vi "Day 14 - Part two.vi"() -> ()   [LabVIEW 2025]
panel:
  out "i":i32
  out "# of sand":i32
  out "cave array":string[][](array[string])
  out "lines array":string[](array[string])
  out "sand pour":i32
  out "Y offset":i32
  out "X":i32
  out "Y":i32
  in  "test":bool
  in  "test input":string="498,4 -> 498,6 -> 496,6\n503,4 -> 502,4 -> 502,9 -> 494,9"
  in  "input":string="487,45 -> 487,38 -> 487,45 -> 489,45 -> 489,42 -> 489,45 -> 491,45 -> 491,39 -> 491,45 -> 493,45 -> 493,39 -> 493,45\n512,90 -> 512,87 -> 512,90 -> 514,90 -> 514,86 -> 514,90 -> 516,90 -> 516,87 -> 516,90 -> 518,90 -> 518,82 -> 518,90 -> 520,90 -> 520,81 -> 520,90 -> 522,90 -> 522,86 -> 522,90 -> 524,90 -> 524,84 -> 524,90 -> 526,90 -> 526,82 -> 526,90 -> 528,90 -> 528,82 -> 528,90\n494,16 -> 499,16\n512,90 -> 512,87 -> 512,90 -> 514,90 -> 514,86 -> 514,90 -> 516,90 -> 516,87 -> 516,90 -> 518,90 -> 518,82 -> 518,90 -> 520,90 -> 520,81 -> 520,90 -> 522,90 -> 522,86 -> 522,90 -> 524,90 -> 524,84 -> 524,90 -> 526,90 -> 526,82 -> 526,90 -> 528,90 -> 528,82 -> 528,90\n505,57 -> 505,59 -> 498,59 -> 498,66 -> 509,66 -> 509,59 -> 507,59 -> 507,57\n492,52 -> 496,52\n520,165 -> 520,160 -> 520,165 -> 522,165 -> 522,163 -> 522,165 -> 524,165 -> 524,159 -> 524,165 -> 526,165 -> 526,159 -> 526,165 -> 528,165 -> 528,155 -> 528,165\n510,123 -> 515,123\n492,48 -> 496,48\n512,90 -> 512,87 -> 512,90 -> 514,90 -> 514,86 -> 514,90 -> 516,90 -> 516,87 -> 516,90 -> 518,90 -> 518,82 -> 518,90 -> 520,90 -> 520,81 -> 520,90 -> 522,90 -> 522,86 -> 522,90 -> 524,90 -> 524,84 -> 524,90 -> 526,90 -> 526,82 -> 526,90 -> 528,90 -> 528,82 -> 528,90\n512,90 -> 512,87 -> 512,90 -> 514,90 -> 514,86 -> 514,90 -> 516,90 -> 516,87 -> 516,90 -> 518,90 -> 518,82 -> 518,90 -> 520,90 -> 520,81 -> 520,90 -> 522,90 -> 522,86 -> 522,90 -> 524,90 -> 524,84 -> 524,90 -> 526,90 -> 526,82 -> 526,90 -> 528,90 -> 528,82 -> 528,90\n487,45 -> 487,38 -> 487,45 -> 489,45 -> 489,42 -> 489,45 -> 491,45 -> 491,39 -> 491,45 -> 493,45 -> 493,39 -> 493,45\n501,54 -> 505,54\n513,120 -> 518,120\n502,138 -> 502,141 -> 498,141 -> 498,145 -> 514,145 -> 514,141 -> 507,141 -> 507,138\n483,54 -> 487,54\n505,57 -> 505,59 -> 498,59 -> 498,66 -> 509,66 -> 509,59 -> 507,59 -> 507,57\n508,103 -> 508,93 -> 508,103 -> 510,103 -> 510,101 -> 510,103 -> 512,103 -> 512,96 -> 512,103\n512,106 -> 512,108 -> 505,108 -> 505,114 -> 518,114 -> 518,108 -> 516,108 -> 516,106\n532,129 -> 537,129\n501,16 -> 506,16\n508,103 -> 508,93 -> 508,103 -> 510,103 -> 510,101 -> 510,103 -> 512,103 -> 512,96 -> 512,103\n502,138 -> 502,141 -> 498,141 -> 498,145 -> 514,145 -> 514,141 -> 507,141 -> 507,138\n520,120 -> 525,120\n489,50 -> 493,50\n498,19 -> 503,19\n505,151 -> 505,152 -> 518,152 -> 518,151\n510,73 -> 514,73\n516,77 -> 520,77\n487,45 -> 487,38 -> 487,45 -> 489,45 -> 489,42 -> 489,45 -> 491,45 -> 491,39 -> 491,45 -> 493,45 -> 493,39 -> 493,45\n520,165 -> 520,160 -> 520,165 -> 522,165 -> 522,163 -> 522,165 -> 524,165 -> 524,159 -> 524,165 -> 526,165 -> 526,159 -> 526,165 -> 528,165 -> 528,155 -> 528,165\n512,90 -> 512,87 -> 512,90 -> 514,90 -> 514,86 -> 514,90 -> 516,90 -> 516,87 -> 516,90 -> 518,90 -> 518,82 -> 518,90 -> 520,90 -> 520,81 -> 520,90 -> 522,90 -> 522,86 -> 522,90 -> 524,90 -> 524,84 -> 524,90 -> 526,90 -> 526,82 -> 526,90 -> 528,90 -> 528,82 -> 528,90\n511,129 -> 516,129\n512,90 -> 512,87 -> 512,90 -> 514,90 -> 514,86 -> 514,90 -> 516,90 -> 516,87 -> 516,90 -> 518,90 -> 518,82 -> 518,90 -> 520,90 -> 520,81 -> 520,90 -> 522,90 -> 522,86 -> 522,90 -> 524,90 -> 524,84 -> 524,90 -> 526,90 -> 526,82 -> 526,90 -> 528,90 -> 528,82 -> 528,90\n520,165 -> 520,160 -> 520,165 -> 522,165 -> 522,163 -> 522,165 -> 524,165 -> 524,159 -> 524,165 -> 526,165 -> 526,159 -> 526,165 -> 528,165 -> 528,155 -> 528,165\n512,90 -> 512,87 -> 512,90 -> 514,90 -> 514,86 -> 514,90 -> 516,90 -> 516,87 -> 516,90 -> 518,90 -> 518,82 -> 518,90 -> 520,90 -> 520,81 -> 520,90 -> 522,90 -> 522,86 -> 522,90 -> 524,90 -> 524,84 -> 524,90 -> 526,90 -> 526,82 -> 526,90 -> 528,90 -> 528,82 -> 528,90\n524,123 -> 529,123\n512,90 -> 512,87 -> 512,90 -> 514,90 -> 514,86 -> 514,90 -> 516,90 -> 516,87 -> 516,90 -> 518,90 -> 518,82 -> 518,90 -> 520,90 -> 520,81 -> 520,90 -> 522,90 -> 522,86 -> 522,90 -> 524,90 -> 524,84 -> 524,90 -> 526,90 -> 526,82 -> 526,90 -> 528,90 -> 528,82 -> 528,90\n505,57 -> 505,59 -> 498,59 -> 498,66 -> 509,66 -> 509,59 -> 507,59 -> 507,57\n487,45 -> 487,38 -> 487,45 -> 489,45 -> 489,42 -> 489,45 -> 491,45 -> 491,39 -> 491,45 -> 493,45 -> 493,39 -> 493,45\n520,165 -> 520,160 -> 520,165 -> 522,165 -> 522,163 -> 522,165 -> 524,165 -> 524,159 -> 524,165 -> 526,165 -> 526,159 -> 526,165 -> 528,165 -> 528,155 -> 528,165\n512,90 -> 512,87 -> 512,90 -> 514,90 -> 514,86 -> 514,90 -> 516,90 -> 516,87 -> 516,90 -> 518,90 -> 518,82 -> 518,90 -> 520,90 -> 520,81 -> 520,90 -> 522,90 -> 522,86 -> 522,90 -> 524,90 -> 524,84 -> 524,90 -> 526,90 -> 526,82 -> 526,90 -> 528,90 -> 528,82 -> 528,90\n507,75 -> 511,75\n495,22 -> 495,25 -> 492,25 -> 492,32 -> 501,32 -> 501,25 -> 499,25 -> 499,22\n514,149 -> 524,149 -> 524,148\n512,90 -> 512,87 -> 512,90 -> 514,90 -> 514,86 -> 514,90 -> 516,90 -> 516,87 -> 516,90 -> 518,90 -> 518,82 -> 518,90 -> 520,90 -> 520,81 -> 520,90 -> 522,90 -> 522,86 -> 522,90 -> 524,90 -> 524,84 -> 524,90 -> 526,90 -> 526,82 -> 526,90 -> 528,90 -> 528,82 -> 528,90\n504,129 -> 509,129\n487,45 -> 487,38 -> 487,45 -> 489,45 -> 489,42 -> 489,45 -> 491,45 -> 491,39 -> 491,45 -> 493,45 -> 493,39 -> 493,45\n520,165 -> 520,160 -> 520,165 -> 522,165 -> 522,163 -> 522,165 -> 524,165 -> 524,159 -> 524,165 -> 526,165 -> 526,159 -> 526,165 -> 528,165 -> 528,155 -> 528,165\n512,90 -> 512,87 -> 512,90 -> 514,90 -> 514,86 -> 514,90 -> 516,90 -> 516,87 -> 516,90 -> 518,90 -> 518,82 -> 518,90 -> 520,90 -> 520,81 -> 520,90 -> 522,90 -> 522,86 -> 522,90 -> 524,90 -> 524,84 -> 524,90 -> 526,90 -> 526,82 -> 526,90 -> 528,90 -> 528,82 -> 528,90\n508,103 -> 508,93 -> 508,103 -> 510,103 -> 510,101 -> 510,103 -> 512,103 -> 512,96 -> 512,103\n504,77 -> 508,77\n495,22 -> 495,25 -> 492,25 -> 492,32 -> 501,32 -> 501,25 -> 499,25 -> 499,22\n516,117 -> 521,117\n514,149 -> 524,149 -> 524,148\n512,90 -> 512,87 -> 512,90 -> 514,90 -> 514,86 -> 514,90 -> 516,90 -> 516,87 -> 516,90 -> 518,90 -> 518,82 -> 518,90 -> 520,90 -> 520,81 -> 520,90 -> 522,90 -> 522,86 -> 522,90 -> 524,90 -> 524,84 -> 524,90 -> 526,90 -> 526,82 -> 526,90 -> 528,90 -> 528,82 -> 528,90\n495,22 -> 495,25 -> 492,25 -> 492,32 -> 501,32 -> 501,25 -> 499,25 -> 499,22\n502,138 -> 502,141 -> 498,141 -> 498,145 -> 514,145 -> 514,141 -> 507,141 -> 507,138\n512,106 -> 512,108 -> 505,108 -> 505,114 -> 518,114 -> 518,108 -> 516,108 -> 516,106\n505,57 -> 505,59 -> 498,59 -> 498,66 -> 509,66 -> 509,59 -> 507,59 -> 507,57\n508,103 -> 508,93 -> 508,103 -> 510,103 -> 510,101 -> 510,103 -> 512,103 -> 512,96 -> 512,103\n508,103 -> 508,93 -> 508,103 -> 510,103 -> 510,101 -> 510,103 -> 512,103 -> 512,96 -> 512,103\n507,126 -> 512,126\n513,75 -> 517,75\n512,90 -> 512,87 -> 512,90 -> 514,90 -> 514,86 -> 514,90 -> 516,90 -> 516,87 -> 516,90 -> 518,90 -> 518,82 -> 518,90 -> 520,90 -> 520,81 -> 520,90 -> 522,90 -> 522,86 -> 522,90 -> 524,90 -> 524,84 -> 524,90 -> 526,90 -> 526,82 -> 526,90 -> 528,90 -> 528,82 -> 528,90\n502,138 -> 502,141 -> 498,141 -> 498,145 -> 514,145 -> 514,141 -> 507,141 -> 507,138\n505,151 -> 505,152 -> 518,152 -> 518,151\n510,77 -> 514,77\n528,126 -> 533,126\n520,165 -> 520,160 -> 520,165 -> 522,165 -> 522,163 -> 522,165 -> 524,165 -> 524,159 -> 524,165 -> 526,165 -> 526,159 -> 526,165 -> 528,165 -> 528,155 -> 528,165\n512,106 -> 512,108 -> 505,108 -> 505,114 -> 518,114 -> 518,108 -> 516,108 -> 516,106\n487,45 -> 487,38 -> 487,45 -> 489,45 -> 489,42 -> 489,45 -> 491,45 -> 491,39 -> 491,45 -> 493,45 -> 493,39 -> 493,45\n487,45 -> 487,38 -> 487,45 -> 489,45 -> 489,42 -> 489,45 -> 491,45 -> 491,39 -> 491,45 -> 493,45 -> 493,39 -> 493,45\n518,129 -> 523,129\n505,57 -> 505,59 -> 498,59 -> 498,66 -> 509,66 -> 509,59 -> 507,59 -> 507,57\n495,22 -> 495,25 -> 492,25 -> 492,32 -> 501,32 -> 501,25 -> 499,25 -> 499,22\n512,90 -> 512,87 -> 512,90 -> 514,90 -> 514,86 -> 514,90 -> 516,90 -> 516,87 -> 516,90 -> 518,90 -> 518,82 -> 518,90 -> 520,90 -> 520,81 -> 520,90 -> 522,90 -> 522,86 -> 522,90 -> 524,90 -> 524,84 -> 524,90 -> 526,90 -> 526,82 -> 526,90 -> 528,90 -> 528,82 -> 528,90\n512,90 -> 512,87 -> 512,90 -> 514,90 -> 514,86 -> 514,90 -> 516,90 -> 516,87 -> 516,90 -> 518,90 -> 518,82 -> 518,90 -> 520,90 -> 520,81 -> 520,90 -> 522,90 -> 522,86 -> 522,90 -> 524,90 -> 524,84 -> 524,90 -> 526,90 -> 526,82 -> 526,90 -> 528,90 -> 528,82 -> 528,90\n487,45 -> 487,38 -> 487,45 -> 489,45 -> 489,42 -> 489,45 -> 491,45 -> 491,39 -> 491,45 -> 493,45 -> 493,39 -> 493,45\n491,19 -> 496,19\n505,19 -> 510,19\n520,165 -> 520,160 -> 520,165 -> 522,165 -> 522,163 -> 522,165 -> 524,165 -> 524,159 -> 524,165 -> 526,165 -> 526,159 -> 526,165 -> 528,165 -> 528,155 -> 528,165\n508,103 -> 508,93 -> 508,103 -> 510,103 -> 510,101 -> 510,103 -> 512,103 -> 512,96 -> 512,103\n506,135 -> 517,135 -> 517,134\n487,45 -> 487,38 -> 487,45 -> 489,45 -> 489,42 -> 489,45 -> 491,45 -> 491,39 -> 491,45 -> 493,45 -> 493,39 -> 493,45\n506,135 -> 517,135 -> 517,134\n520,165 -> 520,160 -> 520,165 -> 522,165 -> 522,163 -> 522,165 -> 524,165 -> 524,159 -> 524,165 -> 526,165 -> 526,159 -> 526,165 -> 528,165 -> 528,155 -> 528,165\n487,45 -> 487,38 -> 487,45 -> 489,45 -> 489,42 -> 489,45 -> 491,45 -> 491,39 -> 491,45 -> 493,45 -> 493,39 -> 493,45\n512,106 -> 512,108 -> 505,108 -> 505,114 -> 518,114 -> 518,108 -> 516,108 -> 516,106\n512,90 -> 512,87 -> 512,90 -> 514,90 -> 514,86 -> 514,90 -> 516,90 -> 516,87 -> 516,90 -> 518,90 -> 518,82 -> 518,90 -> 520,90 -> 520,81 -> 520,90 -> 522,90 -> 522,86 -> 522,90 -> 524,90 -> 524,84 -> 524,90 -> 526,90 -> 526,82 -> 526,90 -> 528,90 -> 528,82 -> 528,90\n520,165 -> 520,160 -> 520,165 -> 522,165 -> 522,163 -> 522,165 -> 524,165 -> 524,159 -> 524,165 -> 526,165 -> 526,159 -> 526,165 -> 528,165 -> 528,155 -> 528,165\n497,13 -> 502,13\n489,54 -> 493,54\n512,90 -> 512,87 -> 512,90 -> 514,90 -> 514,86 -> 514,90 -> 516,90 -> 516,87 -> 516,90 -> 518,90 -> 518,82 -> 518,90 -> 520,90 -> 520,81 -> 520,90 -> 522,90 -> 522,86 -> 522,90 -> 524,90 -> 524,84 -> 524,90 -> 526,90 -> 526,82 -> 526,90 -> 528,90 -> 528,82 -> 528,90\n512,106 -> 512,108 -> 505,108 -> 505,114 -> 518,114 -> 518,108 -> 516,108 -> 516,106\n505,69 -> 505,70 -> 511,70 -> 511,69\n487,45 -> 487,38 -> 487,45 -> 489,45 -> 489,42 -> 489,45 -> 491,45 -> 491,39 -> 491,45 -> 493,45 -> 493,39 -> 493,45\n502,138 -> 502,141 -> 498,141 -> 498,145 -> 514,145 -> 514,141 -> 507,141 -> 507,138\n520,165 -> 520,160 -> 520,165 -> 522,165 -> 522,163 -> 522,165 -> 524,165 -> 524,159 -> 524,165 -> 526,165 -> 526,159 -> 526,165 -> 528,165 -> 528,155 -> 528,165\n512,106 -> 512,108 -> 505,108 -> 505,114 -> 518,114 -> 518,108 -> 516,108 -> 516,106\n512,90 -> 512,87 -> 512,90 -> 514,90 -> 514,86 -> 514,90 -> 516,90 -> 516,87 -> 516,90 -> 518,90 -> 518,82 -> 518,90 -> 520,90 -> 520,81 -> 520,90 -> 522,90 -> 522,86 -> 522,90 -> 524,90 -> 524,84 -> 524,90 -> 526,90 -> 526,82 -> 526,90 -> 528,90 -> 528,82 -> 528,90\n520,165 -> 520,160 -> 520,165 -> 522,165 -> 522,163 -> 522,165 -> 524,165 -> 524,159 -> 524,165 -> 526,165 -> 526,159 -> 526,165 -> 528,165 -> 528,155 -> 528,165\n525,129 -> 530,129\n512,90 -> 512,87 -> 512,90 -> 514,90 -> 514,86 -> 514,90 -> 516,90 -> 516,87 -> 516,90 -> 518,90 -> 518,82 -> 518,90 -> 520,90 -> 520,81 -> 520,90 -> 522,90 -> 522,86 -> 522,90 -> 524,90 -> 524,84 -> 524,90 -> 526,90 -> 526,82 -> 526,90 -> 528,90 -> 528,82 -> 528,90\n512,90 -> 512,87 -> 512,90 -> 514,90 -> 514,86 -> 514,90 -> 516,90 -> 516,87 -> 516,90 -> 518,90 -> 518,82 -> 518,90 -> 520,90 -> 520,81 -> 520,90 -> 522,90 -> 522,86 -> 522,90 -> 524,90 -> 524,84 -> 524,90 -> 526,90 -> 526,82 -> 526,90 -> 528,90 -> 528,82 -> 528,90\n505,151 -> 505,152 -> 518,152 -> 518,151\n495,22 -> 495,25 -> 492,25 -> 492,32 -> 501,32 -> 501,25 -> 499,25 -> 499,22\n521,126 -> 526,126\n512,106 -> 512,108 -> 505,108 -> 505,114 -> 518,114 -> 518,108 -> 516,108 -> 516,106\n495,50 -> 499,50\n495,54 -> 499,54\n502,138 -> 502,141 -> 498,141 -> 498,145 -> 514,145 -> 514,141 -> 507,141 -> 507,138\n512,90 -> 512,87 -> 512,90 -> 514,90 -> 514,86 -> 514,90 -> 516,90 -> 516,87 -> 516,90 -> 518,90 -> 518,82 -> 518,90 -> 520,90 -> 520,81 -> 520,90 -> 522,90 -> 522,86 -> 522,90 -> 524,90 -> 524,84 -> 524,90 -> 526,90 -> 526,82 -> 526,90 -> 528,90 -> 528,82 -> 528,90\n508,103 -> 508,93 -> 508,103 -> 510,103 -> 510,101 -> 510,103 -> 512,103 -> 512,96 -> 512,103\n512,90 -> 512,87 -> 512,90 -> 514,90 -> 514,86 -> 514,90 -> 516,90 -> 516,87 -> 516,90 -> 518,90 -> 518,82 -> 518,90 -> 520,90 -> 520,81 -> 520,90 -> 522,90 -> 522,86 -> 522,90 -> 524,90 -> 524,84 -> 524,90 -> 526,90 -> 526,82 -> 526,90 -> 528,90 -> 528,82 -> 528,90\n508,103 -> 508,93 -> 508,103 -> 510,103 -> 510,101 -> 510,103 -> 512,103 -> 512,96 -> 512,103\n512,90 -> 512,87 -> 512,90 -> 514,90 -> 514,86 -> 514,90 -> 516,90 -> 516,87 -> 516,90 -> 518,90 -> 518,82 -> 518,90 -> 520,90 -> 520,81 -> 520,90 -> 522,90 -> 522,86 -> 522,90 -> 524,90 -> 524,84 -> 524,90 -> 526,90 -> 526,82 -> 526,90 -> 528,90 -> 528,82 -> 528,90\n495,22 -> 495,25 -> 492,25 -> 492,32 -> 501,32 -> 501,25 -> 499,25 -> 499,22\n498,52 -> 502,52\n517,123 -> 522,123\n514,126 -> 519,126\n512,90 -> 512,87 -> 512,90 -> 514,90 -> 514,86 -> 514,90 -> 516,90 -> 516,87 -> 516,90 -> 518,90 -> 518,82 -> 518,90 -> 520,90 -> 520,81 -> 520,90 -> 522,90 -> 522,86 -> 522,90 -> 524,90 -> 524,84 -> 524,90 -> 526,90 -> 526,82 -> 526,90 -> 528,90 -> 528,82 -> 528,90\n512,90 -> 512,87 -> 512,90 -> 514,90 -> 514,86 -> 514,90 -> 516,90 -> 516,87 -> 516,90 -> 518,90 -> 518,82 -> 518,90 -> 520,90 -> 520,81 -> 520,90 -> 522,90 -> 522,86 -> 522,90 -> 524,90 -> 524,84 -> 524,90 -> 526,90 -> 526,82 -> 526,90 -> 528,90 -> 528,82 -> 528,90\n495,22 -> 495,25 -> 492,25 -> 492,32 -> 501,32 -> 501,25 -> 499,25 -> 499,22\n505,69 -> 505,70 -> 511,70 -> 511,69\n520,165 -> 520,160 -> 520,165 -> 522,165 -> 522,163 -> 522,165 -> 524,165 -> 524,159 -> 524,165 -> 526,165 -> 526,159 -> 526,165 -> 528,165 -> 528,155 -> 528,165\n512,90 -> 512,87 -> 512,90 -> 514,90 -> 514,86 -> 514,90 -> 516,90 -> 516,87 -> 516,90 -> 518,90 -> 518,82 -> 518,90 -> 520,90 -> 520,81 -> 520,90 -> 522,90 -> 522,86 -> 522,90 -> 524,90 -> 524,84 -> 524,90 -> 526,90 -> 526,82 -> 526,90 -> 528,90 -> 528,82 -> 528,90\n520,165 -> 520,160 -> 520,165 -> 522,165 -> 522,163 -> 522,165 -> 524,165 -> 524,159 -> 524,165 -> 526,165 -> 526,159 -> 526,165 -> 528,165 -> 528,155 -> 528,165\n505,57 -> 505,59 -> 498,59 -> 498,66 -> 509,66 -> 509,59 -> 507,59 -> 507,57\n520,165 -> 520,160 -> 520,165 -> 522,165 -> 522,163 -> 522,165 -> 524,165 -> 524,159 -> 524,165 -> 526,165 -> 526,159 -> 526,165 -> 528,165 -> 528,155 -> 528,165\n505,69 -> 505,70 -> 511,70 -> 511,69\n505,57 -> 505,59 -> 498,59 -> 498,66 -> 509,66 -> 509,59 -> 507,59 -> 507,57\n502,138 -> 502,141 -> 498,141 -> 498,145 -> 514,145 -> 514,141 -> 507,141 -> 507,138\n486,52 -> 490,52\n"
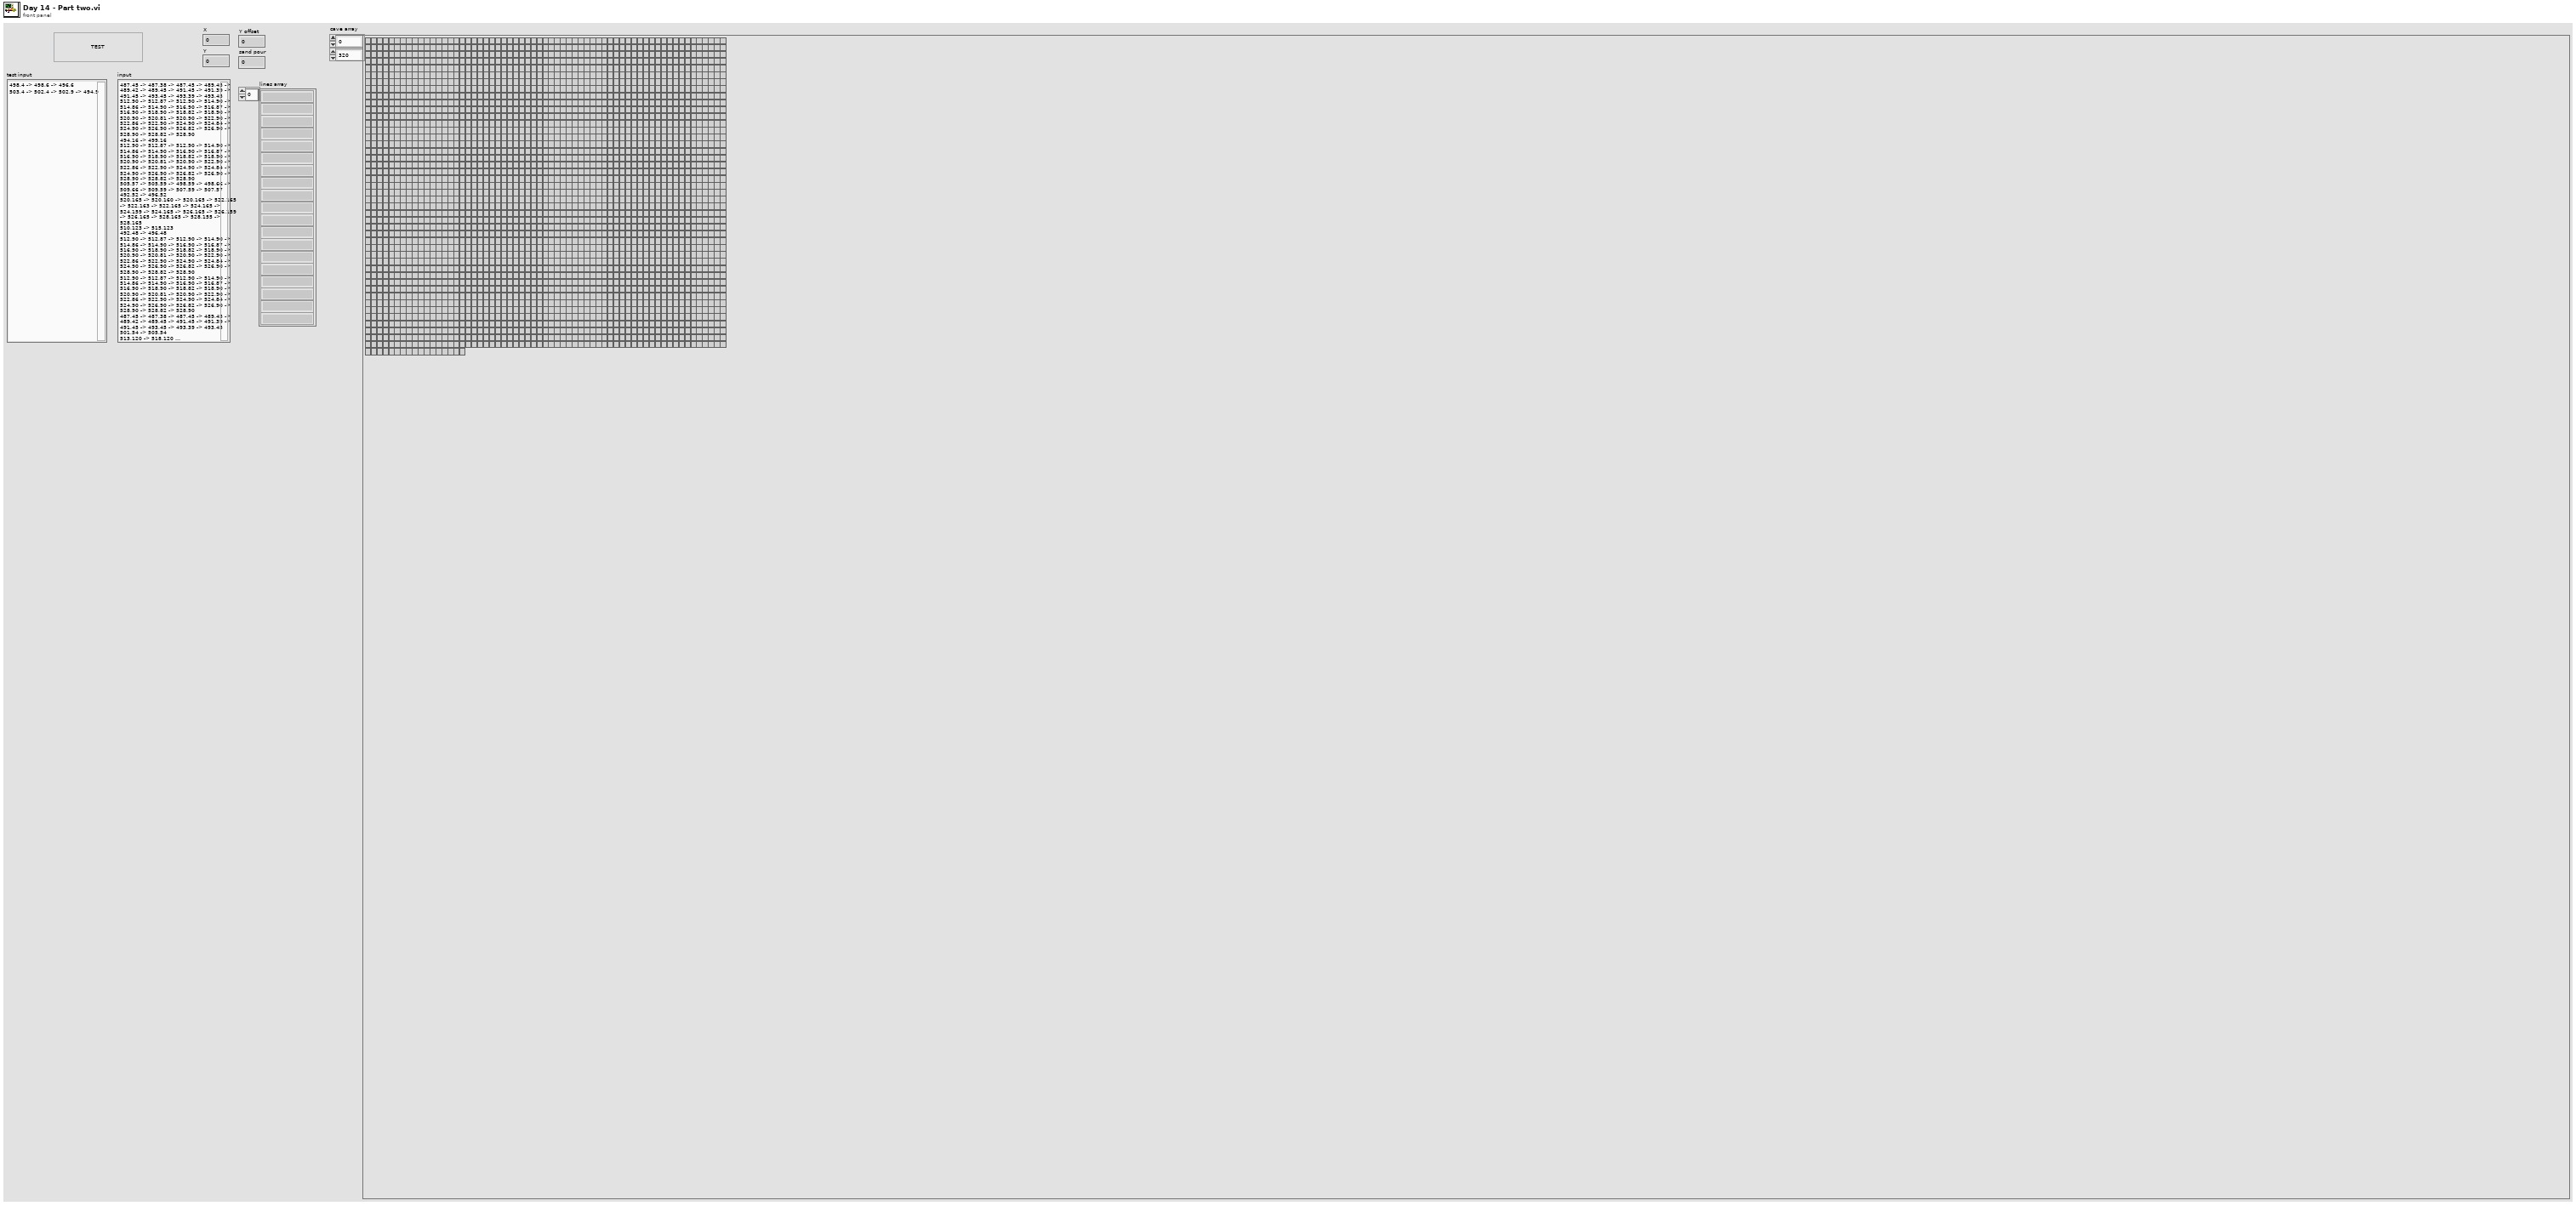
[diagram p1: front panel]
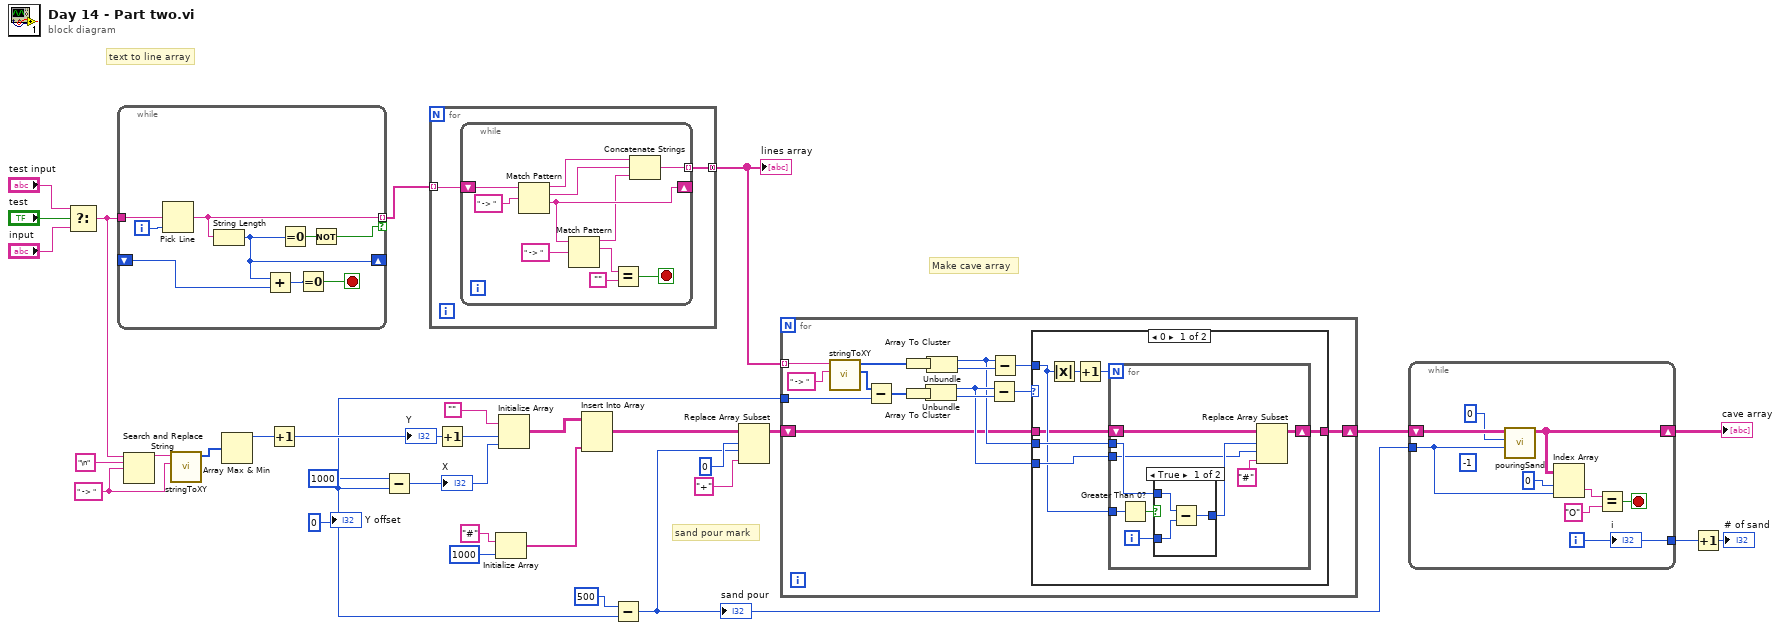
[diagram p0: block diagram]
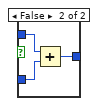
[diagram p2: hidden frame]
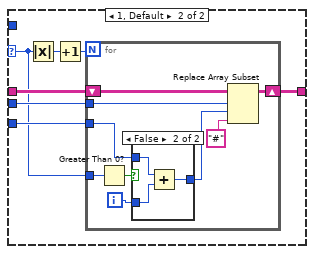
[diagram p3: hidden frame]
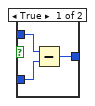
[diagram p4: hidden frame]
diagram:
  w9 = 0
  w25 = " -> " ("delimiter")
  # "Make cave array"
  # "sand pour mark"
  # "text to line array"
  n1 = Select(t="test input", s="test", f="input") -> (s? t:f=w28:string)
  n2 = while {
    tunnel: w28 -> [w39]
    tunnel: [w32] -> w22 mode=indexing if=w38
    shift-right: [w35] -> _
    shift-left: _ -> [w36]
    i -> [w40]
    stop <- w33 stop-if-true
    n3 = Pick Line(multi-line string=w39, line index=w40) -> (output string=w32:string)  [unwired: 1 in]
    n4 = String Length(string=w32) -> (length=w35:i32)
    n5 = Add(x=w35, y=w36) -> (x+y=w37:i32)
    n6 = Equal To 0?(x=w35) -> (x = 0?=w34:bool)
    n7 = Equal To 0?(x=w37) -> (x = 0?=w33:bool)
    n8 = Not(x=w34) -> (.not. x?=w38:bool)
  }
  n9 = Search and Replace String(input string=w28, search string="\n", replace string=w25) -> (result string=w27:string)  [unwired: 5 in, 3 out]
  n10 = call "stringToXY.vi"("delimiter"=w25, "string"=w27) -> ("Y"=w15:i32[])  [unwired: 8 in, 1 out]
  n11 = Array Max & Min(array=w15) -> (max value=w20:i32)  [unwired: 3 out]
  n12 = Increment(x=w20) -> (x+1=w13:i32)
  "Y" <- w13
  n13 = Subtract(x=1000, y=w9) -> (x-y=w18:i32)
  "X" <- w18
  n14 = for {
    tunnel: w22 -> [w42] mode=indexing
    tunnel: [w41] -> w21 mode=concatenating
    n15 = while {
      shift-right: [w50] -> _
      shift-left: w42 -> [w52]
      tunnel: [w47] -> w41 mode=indexing
      stop <- w44 stop-if-true
      n16 = Match Pattern(string=w52, regular expression=" -> " ("delimiter")) -> (before substring=w49:string, match substring=w48:string, after substring=w50:string)  [unwired: 1 in, 1 out]
      n17 = Match Pattern(string=w50, regular expression=" -> " ("delimiter")) -> (before substring=w43:string, match substring=w45:string)  [unwired: 1 in, 2 out]
      n18 = Equal?(x=w45, y="") -> (x = y?=w44:bool)
      n19 = Concatenate Strings(w49, w48, w43) -> (w47:string)
    }
  }
  "lines array" <- w21
  n20 = Increment(x=w13) -> (x+1=w10:i32)
  n21 = Initialize Array("#", 1000 ("dimension size")) -> (w3:string[])
  n22 = Initialize Array("", w10, w18) -> (w4:string[][])
  n23 = Insert Into Array(array=w4, new element=w3) -> (w5:string[][])  [unwired: 2 in]
  n24 = Subtract(x=500, y=w9) -> (x-y=w12:i32)
  "sand pour" <- w12
  n25 = Replace Array Subset(array=w5, new element="+" ("new element/subarray"), index (row)=0 ("index (col)"), index (col)=w12) -> (w16:string[][])
  n26 = for {
    tunnel: w21 -> [w57] mode=indexing
    shift-right: [w60] -> w14
    shift-left: w16 -> [w59]
    tunnel: w9 -> [w56]
    n27 = call "stringToXY.vi"("delimiter"=" -> ", "string"=w57) -> ("X"=w55:i32[], "Y"=w54:i32[])  [unwired: 8 in]
    n28 = Subtract(x=w55, y=w56) -> (x-y=w58:i32[])
    n29 = Array To Cluster(array=w54) -> (cluster=w67:cluster{"Y[0]":i32, "Y[1]":i32})
    n30 = Array To Cluster(array=w58) -> (cluster=w68:cluster{"[0]":i32, "[1]":i32})
    n31 = Unbundle(w68) -> ("[0]"=w62:i32, "[1]"=w66:i32)
    n32 = Unbundle(w67) -> ("Y[0]"=w61:i32, "Y[1]"=w64:i32)
    n33 = Subtract(x=w62, y=w66) -> (x-y=w65:i32)
    n34 = Subtract(x=w61, y=w64) -> (x-y=w63:i32)
    n35 = case shown="0" w65 {
      selector: w65 -> [_ w93]
      tunnel: w63 -> [w73 _]
      tunnel: w62 -> [w75 w97]
      tunnel: w61 -> [w74 w96]
      tunnel: [w72 w95] -> w60
      tunnel: w59 -> [w71 w94]
      frame 0 {
        n36 = Absolute Value(x=w73) -> (abs(x)=w76:i32)
        n37 = Increment(x=w76) -> (x+1=w70:i32)
        n38 = for {
          N: w70 -> [_]
          tunnel: w75 -> [w77]
          tunnel: w74 -> [w84]
          tunnel: w73 -> [w85]
          shift-right: [w81] -> w72
          shift-left: w71 -> [w82]
          i -> [w83]
          n39 = Greater Than 0?(x=w85) -> (x > 0?=w80:bool)
          n40 = case shown="True" w80 {
            tunnel: w84 -> [w88 w91]
            tunnel: w83 -> [w87 w90]
            tunnel: [w86 w89] -> w79
            frame True {
              n41 = Subtract(x=w88, y=w87) -> (x-y=w86:i32)
            }
            frame False {
              n42 = Add(x=w91, y=w90) -> (x+y=w89:i32)
            }
          }
          n43 = Replace Array Subset(array=w82, new element="#" ("new element/subarray"), index (row)=w79, index (col)=w77) -> (w81:string[][])
        }
      }
      frame 1, Default {
        n44 = Absolute Value(x=w93) -> (abs(x)=w98:i32)
        n45 = Increment(x=w98) -> (x+1=w92:i32)
        n46 = for {
          N: w92 -> [_]
          tunnel: w97 -> [w102]
          tunnel: w96 -> [w100]
          tunnel: w93 -> [w106]
          shift-right: [w103] -> w95
          shift-left: w94 -> [w104]
          i -> [w105]
          n47 = Greater Than 0?(x=w106) -> (x > 0?=w107:bool)
          n48 = case shown="False" w107 {
            tunnel: w102 -> [w110 w113]
            tunnel: w105 -> [w109 w112]
            tunnel: [w108 w111] -> w99
            frame True {
              n49 = Subtract(x=w110, y=w109) -> (x-y=w108:i32)
            }
            frame False {
              n50 = Add(x=w113, y=w112) -> (x+y=w111:i32)
            }
          }
          n51 = Replace Array Subset(array=w104, new element="#" ("new element/subarray"), index (row)=w100, index (col)=w99) -> (w103:string[][])
        }
      }
    }
  }
  n52 = while {
    tunnel: w12 -> [w119]
    shift-right: [w115] -> w1
    shift-left: w14 -> [w122]
    tunnel: [w114] -> w11
    i -> [w114]
    stop <- w116 stop-if-true
    (unwired) -1 ("Y max")
    n53 = call "pouringSand.vi"("sand pour"=w119, "Y"=0, "cave"=w122) -> ("cave"=w115:string[][])  [unwired: 7 in, 1 out]
    n54 = Index Array(array=w115, index (row)=0, index (col)=w119) -> (element=w118:string)
    n55 = Equal?(x=w118, y="O") -> (x = y?=w116:bool)
    "i" <- w114
  }
  "cave array" <- w1
  n56 = Increment(x=w11) -> (x+1=→"# of sand":i32)
  "Y offset" <- w9
